vi "constructor.vi"(8 "error in (no error)":errorcluster, 10 "Camera":string) -> (0 "error out":errorcluster, 3 "Camera out":refnum<class "Camera.lvclass">)   [LabVIEW 2011, in "Hardware.lvlib" / "Channels.lvlib" / "Camera.lvclass"]
uses:
  Camera.lvclass
  Pixelfly/Pixelfly.lvclass
  ProEM_WinX32/ProEM_WinX32.lvclass
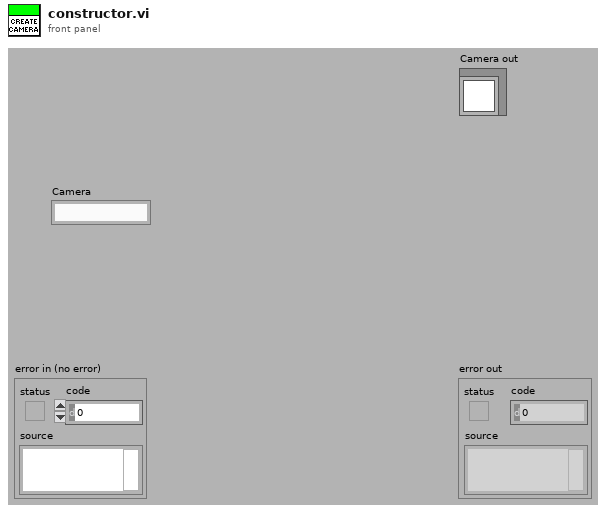
[diagram p1: front panel]
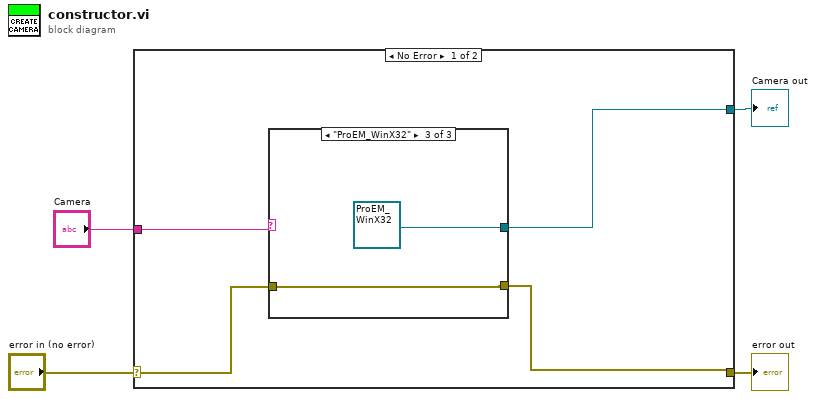
[diagram p0: block diagram]
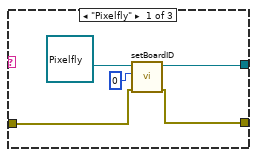
[diagram p2: hidden frame]
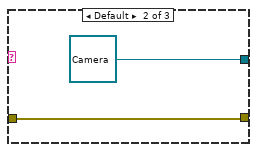
[diagram p3: hidden frame]
diagram:
  n1 = case shown="No Error" "error in (no error)" {
    selector: "error in (no error)" -> [w6 w18]
    tunnel: [w5 w18] -> w3
    tunnel: "Camera" -> [w8 _]
    tunnel: [w7 _] -> w1
    frame No Error {
      n2 = case shown="\"ProEM_WinX32\"" w8 {
        tunnel: [w13 refnum<class "Camera.lvclass"> refnum ("Camera in") refnum<class "ProEM_WinX32.lvclass"> refnum ("Hardware:Channels.lvlib:ProEM_WinX32.lvclass")] -> w7
        tunnel: w6 -> [w10 w14 w16]
        tunnel: [w9 w14 w16] -> w5
        frame "Pixelfly" {
          n3 = call "setBoardID.vi"("error in (no error)"=w10, "boardID"=0, "Pixelfly in"=refnum<class "Pixelfly.lvclass"> refnum ("Hardware:Channels.lvlib:Pixelfly.lvclass")) -> ("error out"=w9:errorcluster, "Pixelfly out"=w13:refnum<class "Pixelfly.lvclass">)  [unwired: 7 in]
        }
        frame Default {
        }
        frame "ProEM_WinX32" {
        }
      }
    }
    frame Error {
    }
  }
  "error out" <- w3
  "Camera out" <- w1
